vi "Length_4.vi"() -> ()   [LabVIEW 2020]
uses:
  Support/Controls/Cmd_Mouse Popup.ctl
  Support/Controls/Clst_Initialize Input.ctl
  Support/Controls/Clst_Result inspec.ctl
  Support/Controls/Cmd_Var Data IO.ctl
  Variables/Global_Cal Info.vi
panel:
  out "최소범위":string
  in  "구분 2":string(combo) caption="재질"
  in  "구분":string(combo)="2급" caption="등급"
  out "단위":string
  out "최대범위":string
  in  "Spec 변경":bool
  in  "Random":bool
  out "Spec":string[][](table)
  out "제목":string
  out "에러 출력":errorcluster
  out "Condition":string[][](table) caption="2. 직선성 시험"
  in  "Measured":string[][](table) caption="지시편차 (μm)"
  out "Load?":bool
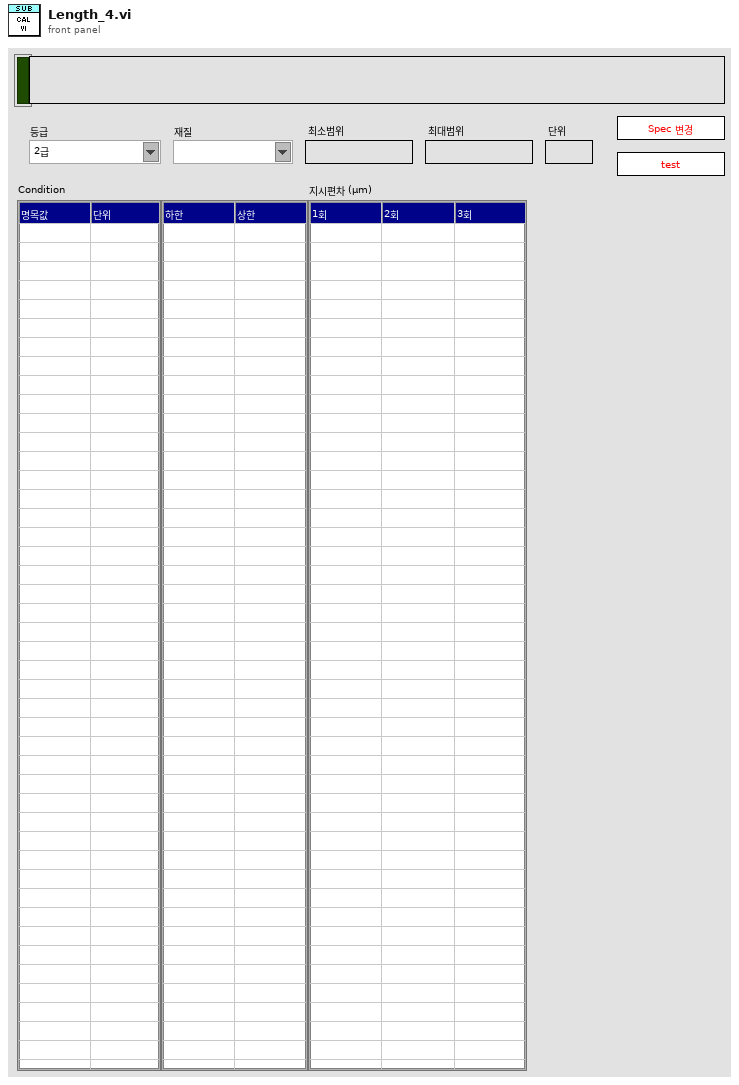
[diagram p1: front panel]
types:
  T1 = typedef "Cmd_Mouse Popup.ctl" = enum16{"활성화", "메뉴선택"}
  T2 = cluster{"Shift":bool, "Ctrl":bool, "Alt":bool, "Cmd":bool, "Opt":bool}
  T3 = typedef "Clst_Initialize Input.ctl" = cluster{"Initialize 1":cluster{"Condition":refnum<vi>[], "Spec":refnum<vi>[], "Measured":refnum<vi>[], "Resolution":refnum<vi>[], "Func_ext":string, "제목":refnum<vi>, "Measured_ADJ":refnum<vi>[]}, "Initialize 2":cluster{"문자열":refnum<vi>[], "콤보박스":refnum<vi>[], "링":refnum<vi>[], "열거형":refnum<vi>[], "테이블":refnum<vi>[], "여러열":refnum<vi>[], "디지털(DBL)":refnum<vi>[], "3D string":refnum<vi>[], "ctrl":refnum<vi>[], "boolean":refnum<vi>[]}}
  T4 = enum8{"Enabled", "Disabled", "Disabled and Grayed Out"}
  T5 = typedef "Clst_Result inspec.ctl" = cluster{"분해능":string, "문자열 1":string, "문자열 2":string, "숫자형 1":i32, "숫자형 2":i32, "숫자형 3":dbl, "문자배열 1D":string[], "문자배열 2D":string[][], "문자배열 3D":string[][][], "문자배열 4D":string[][][][], "불리언 1D":bool[]}
  T6 = typedef "Cmd_Var Data IO.ctl" = enum16{"Condition", "Condition Default", "Condition_Temp", "Resolution", "Resolution Default", "Resolution Old", "Spec", "Spec Default", "Spec Old", "Spec Temp", "Result", "Result2", "Result3", "Result_Temp", "Result_ADJ", "Result_ADJ2", "STD1", "STD2", "STD3", "STD4", "STD5", "STD Temp", "CMC", "CMC Default"}
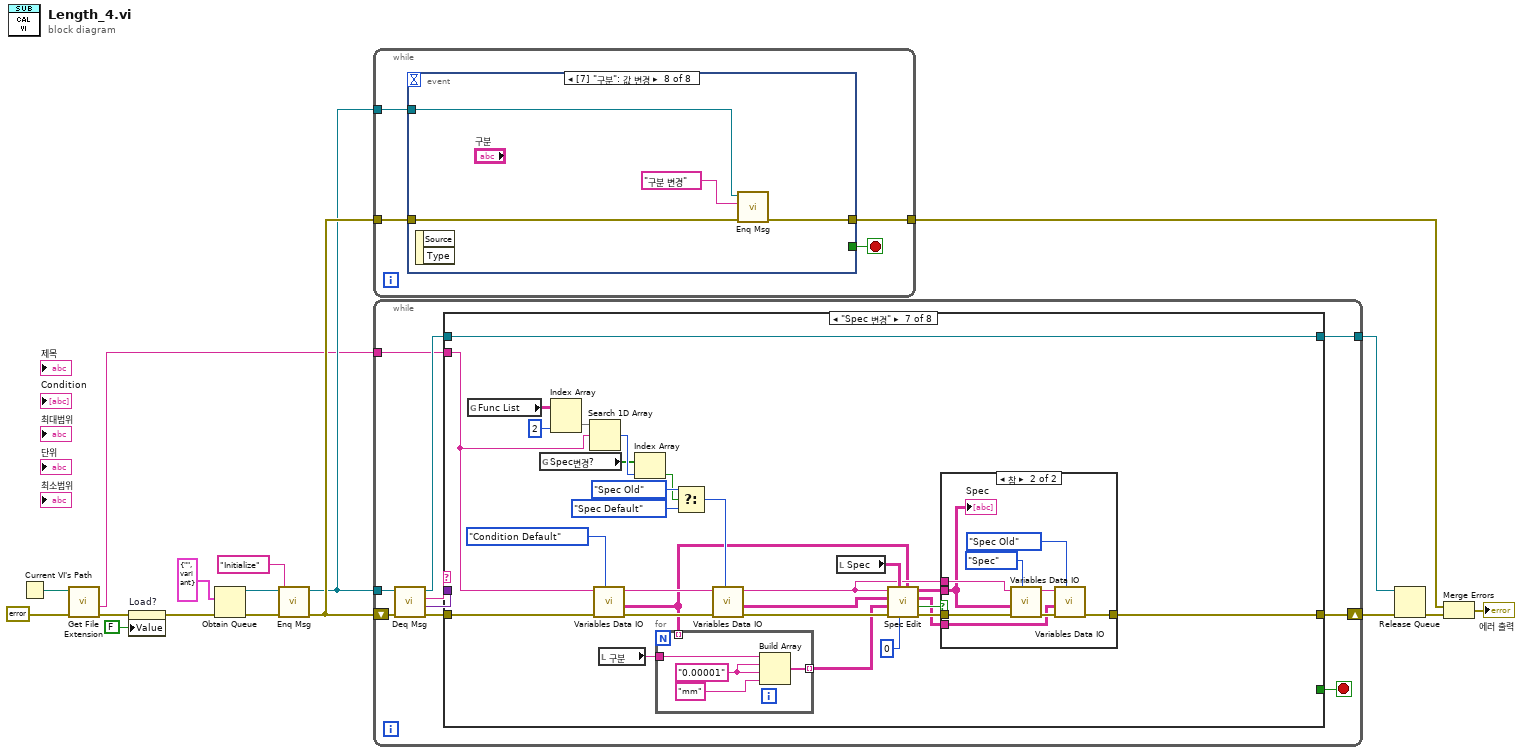
[diagram p0: block diagram]
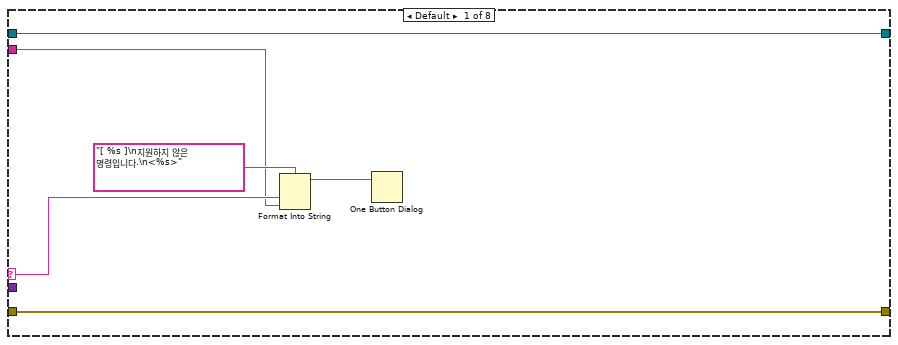
[diagram p2: hidden frame]
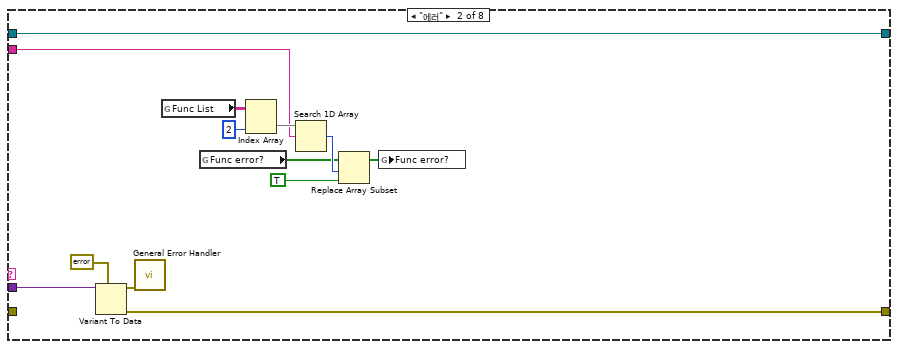
[diagram p3: hidden frame]
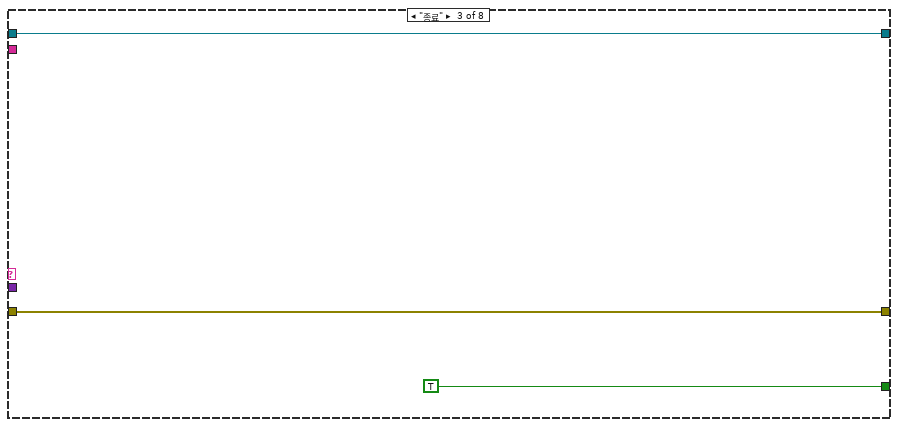
[diagram p4: hidden frame]
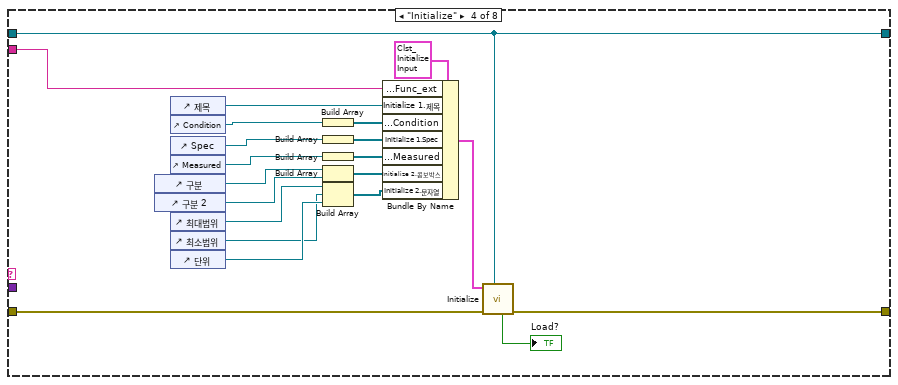
[diagram p5: hidden frame]
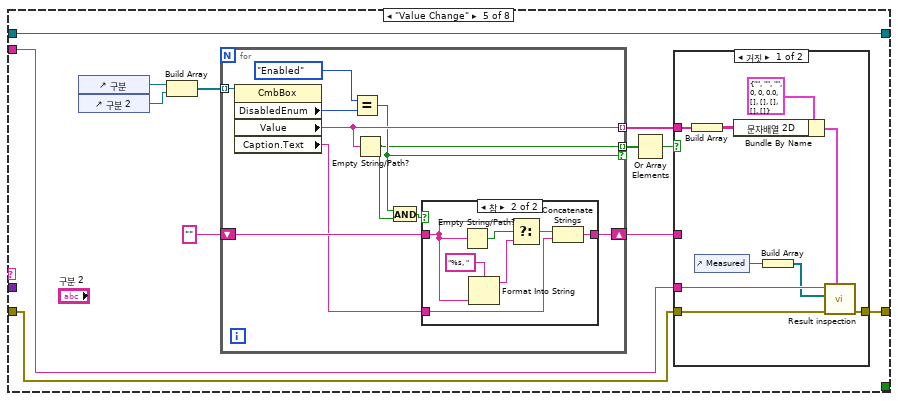
[diagram p6: hidden frame]
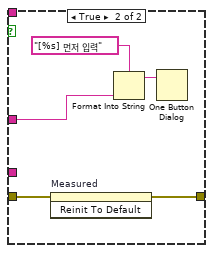
[diagram p8: hidden frame]
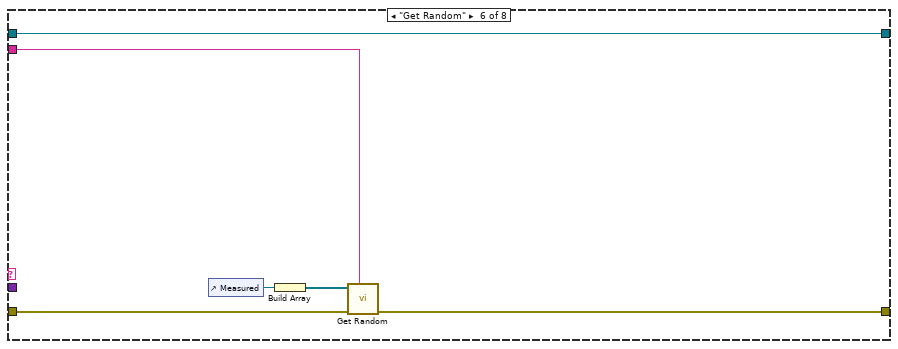
[diagram p9: hidden frame]
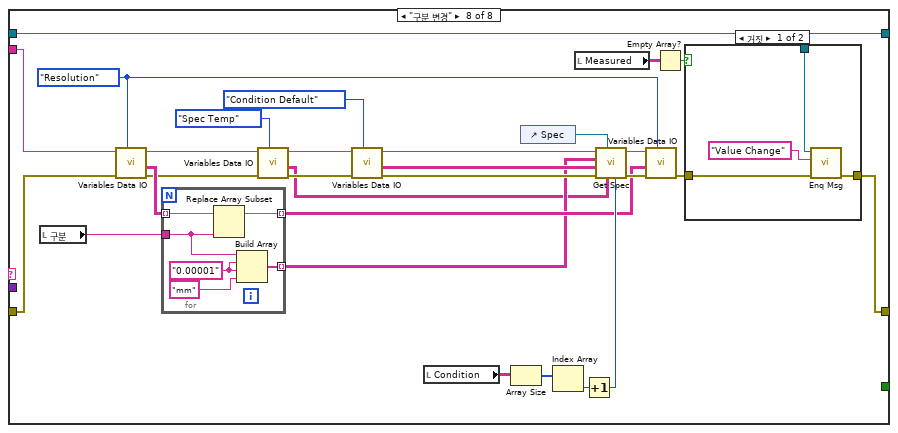
[diagram p11: hidden frame]
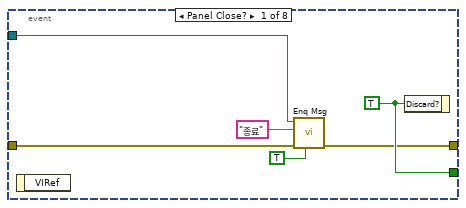
[diagram p13: hidden frame]
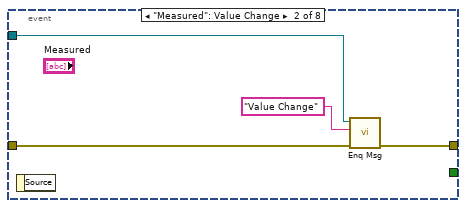
[diagram p14: hidden frame]
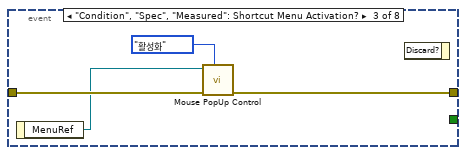
[diagram p15: hidden frame]
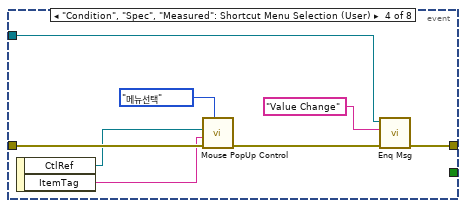
[diagram p16: hidden frame]
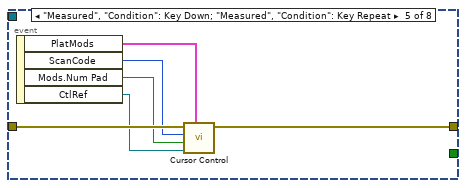
[diagram p17: hidden frame]
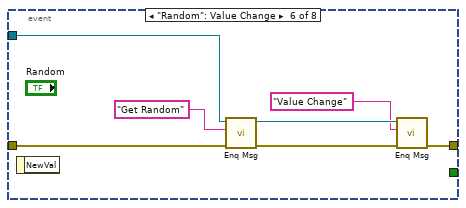
[diagram p18: hidden frame]
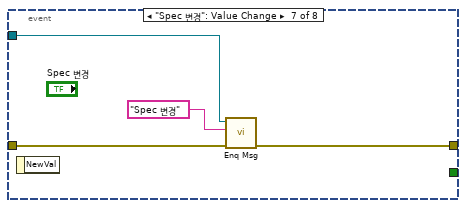
[diagram p19: hidden frame]
diagram:
  n1 = Current VI's Path() -> (path=w5:path)
  n2 = call <vilib>:"Get File Extension.vi"("error in (no error)"=errorcluster {"status"=FALSE, "code"=0, "source"=""} ("에러 상수"), "file"=w5) -> ("error out"=w3:errorcluster, "filename without extension"=w4:string)  [unwired: 5 in, 3 out]
  n3 = property on="Load?" class="Bool (엄격한)"(error in=w3, "Value"=FALSE ("Load?")) -> (error out=w2:errorcluster)  [unwired: 1 in, 1 out]
  n4 = Obtain Queue(element data type=cluster{"메세지":string, "값":variant} {"메세지"="", "값"=variant} ("Message Cluster"), error in (no error)=w2) -> (queue out=w14:refnum<queue>, error out=w16:errorcluster)  [unwired: 3 in, 1 out]
  n5 = call "Enq Msg.vi"("에러 입력(에러 없음)"=w16, "메세지"="Initialize", "큐 입력"=w14) -> ("에러 출력"=w15:errorcluster, "큐 출력"=w12:refnum<queue>)  [unwired: 7 in]
  n6 = while {
    tunnel: w15 -> [w19]
    tunnel: w12 -> [w20]
    tunnel: [w18] -> w9
    stop <- w21 stop-if-true
    n7 = event shown="[7] \"구분\": 값 변경" {
      selector: _ -> [_ _ _ _ _ _ _ _]
      dyn-events: _ -> [_ _ _ _ _ _ _ _]
      timeout: _ -> [_ _ _ _ _ _ _ _]
      tunnel: [w27 _ _ _ _ _ _ _] -> w21
      tunnel: w20 -> [w25 w31 _ w36 _ w54 w58 w61]
      tunnel: w19 -> [w26 w29 w35 w43 w49 w55 w59 w63]
      tunnel: [w23 w30 w34 w37 w48 w50 w57 w62] -> w18
      event Panel Close? {
        w27 = TRUE ("버림?")
        n8 = event-data() -> ()  [unwired: 1 in, 1 out]
        n9 = call "Enq Msg.vi"("우선순위 메시지?"=TRUE, "에러 입력(에러 없음)"=w26, "메세지"="종료", "큐 입력"=w25) -> ("에러 출력"=w23:errorcluster)  [unwired: 6 in, 1 out]
        n10 = event-data("Discard?"=w27) -> ()  [unwired: 1 in, 1 out]
      }
      event "Measured": Value Change {
        n11 = event-data() -> ()  [unwired: 1 in, 1 out]
        n12 = call "Enq Msg.vi"("에러 입력(에러 없음)"=w29, "메세지"="Value Change", "큐 입력"=w31) -> ("에러 출력"=w30:errorcluster)  [unwired: 7 in, 1 out]
      }
      event "Condition", "Spec", "Measured": Shortcut Menu Activation? {
        n13 = event-data() -> ("MenuRef"=w33:refnum<k9>)  [unwired: 1 in]
        n14 = call "Mouse PopUp Control.vi"("type"=Cmd_Mouse_Popup."활성화", "error in"=w35, "메뉴 참조"=w33) -> ("error out"=w34:errorcluster)  [unwired: 8 in]
        n15 = event-data() -> ()  [unwired: 2 in, 1 out]
      }
      event "Condition", "Spec", "Measured": Shortcut Menu Selection (User) {
        n16 = event-data() -> ("CtlRef"=w41:refnum<vi>, "ItemTag"=w40:string)  [unwired: 1 in]
        n17 = call "Mouse PopUp Control.vi"("type"=Cmd_Mouse_Popup."메뉴선택", "error in"=w43, "아이템 태그"=w40, "Tbl 참조 번호"=w41) -> ("error out"=w38:errorcluster)  [unwired: 7 in]
        n18 = call "Enq Msg.vi"("에러 입력(에러 없음)"=w38, "메세지"="Value Change", "큐 입력"=w36) -> ("에러 출력"=w37:errorcluster)  [unwired: 7 in, 1 out]
      }
      event "Measured", "Condition": Key Down; "Measured", "Condition": Key Repeat {
        n19 = event-data() -> ("PlatMods"=w44:T2, "ScanCode"=w47:i16, "Mods.Num Pad"=w46:bool, "CtlRef"=w45:refnum<vi>)  [unwired: 1 in]
        n20 = call "Cursor Control.vi"("플랫폼 조합키"=w44, "참조"=w45, "Num Pad"=w46, "ScanCode"=w47, "error in"=w49) -> ("error out"=w48:errorcluster)  [unwired: 5 in, 1 out]
      }
      event "Random": Value Change {
        n21 = event-data() -> ()  [unwired: 1 in, 1 out]
        n22 = call "Enq Msg.vi"("에러 입력(에러 없음)"=w55, "메세지"="Get Random", "큐 입력"=w54) -> ("에러 출력"=w53:errorcluster, "큐 출력"=w52:refnum<queue>)  [unwired: 7 in]
        n23 = call "Enq Msg.vi"("에러 입력(에러 없음)"=w53, "메세지"="Value Change", "큐 입력"=w52) -> ("에러 출력"=w50:errorcluster)  [unwired: 7 in, 1 out]
      }
      event "Spec 변경": Value Change {
        n24 = event-data() -> ()  [unwired: 1 in, 1 out]
        n25 = call "Enq Msg.vi"("에러 입력(에러 없음)"=w59, "메세지"="Spec 변경", "큐 입력"=w58) -> ("에러 출력"=w57:errorcluster)  [unwired: 7 in, 1 out]
      }
      event "구분": Value Change {
        n26 = event-data() -> ()  [unwired: 1 in, 2 out]
        n27 = call "Enq Msg.vi"("에러 입력(에러 없음)"=w63, "메세지"="구분 변경", "큐 입력"=w61) -> ("에러 출력"=w62:errorcluster)  [unwired: 7 in, 1 out]
      }
    }
  }
  n28 = while {
    shift-right: [w74] -> w11
    shift-left: w15 -> [w73]
    tunnel: w12 -> [w71]
    tunnel: [w66] -> w10
    tunnel: w4 -> [w65]
    stop <- w67 stop-if-true
    n29 = call "Deq Msg.vi"("에러 입력(에러 없음)"=w73, "큐 입력"=w71) -> ("에러 출력"=w72:errorcluster, "값"=w68:variant, "메세지"=w70:string, "큐 출력"=w69:refnum<queue>)  [unwired: 6 in]
    n30 = case shown="\"Spec 변경\"" w70 {
      selector: w70 -> [w76 _ _ _ _ _ _ _]
      tunnel: w72 -> [w80 _ w96 w117 w126 w163 w171 w219]
      tunnel: [w80 w90 w96 w108 w128 w164 w191 w227] -> w74
      tunnel: w69 -> [w79 w89 w94 w104 w129 w167 w195 w226]
      tunnel: w68 -> [_ w91 _ _ _ _ _ _]
      tunnel: [_ _ TRUE ("버림?") _ _ _ _ _] -> w67
      tunnel: [w79 w89 w94 w104 w129 w167 w195 w226] -> w66
      tunnel: w65 -> [w75 w81 _ w105 w127 w162 w172 w220]
      frame Default {
        n31 = Format Into String(format string="[ %s ]\n지원하지 않은 명령입니다.\n<%s>" ("메시지"), w76, w75) -> (resulting string=w77:string)  [unwired: 2 in, 1 out]
        n32 = One Button Dialog(message=w77) -> ()  [unwired: 1 in, 1 out]
      }
      frame "에러" {
        n33 = Variant To Data(type=errorcluster {"status"=FALSE, "code"=0, "source"=""} ("에러 출력"), Variant=w91) -> (data=w93:errorcluster, error out=w90:errorcluster)  [unwired: 1 in]
        n34 = call <vilib>:"General Error Handler.vi"("error in (no error)"=w93) -> ()  [unwired: 10 in, 5 out]
        n35 = global read "Global_Cal Info.vi" "Func List"() -> (w83:string[][])
        n36 = global read "Global_Cal Info.vi" "Func error?"() -> (w86:bool[])
        n37 = Index Array(array=w83, index (col)=2 ("비활성화된 인덱스 (열)")) -> (element=w84:string[])  [unwired: 1 in]
        n38 = Search 1D Array(1D array=w84, element=w81) -> (index of element=w87:i32)  [unwired: 1 in]
        n39 = Replace Array Subset(array=w86, new element=TRUE ("새 원소/부분배열"), index=w87) -> (w88:bool[])
        n40 = global write "Global_Cal Info.vi" "Func error?"(w88) -> ()
      }
      frame "종료" {
      }
      frame "Initialize" {
        n41 = control-ref of="구분"() -> (w100:refnum<vi>)
        n42 = control-ref of="구분 2"() -> (w99:refnum<vi>)
        n43 = control-ref of="제목"() -> (w109:refnum<vi>)
        n44 = control-ref of="Condition"() -> (w114:refnum<vi>)
        n45 = control-ref of="Spec"() -> (w107:refnum<vi>)
        n46 = control-ref of="Measured"() -> (w111:refnum<vi>)
        n47 = control-ref of="최대범위"() -> (w101:refnum<vi>)
        n48 = control-ref of="최소범위"() -> (w97:refnum<vi>)
        n49 = control-ref of="단위"() -> (w103:refnum<vi>)
        n50 = Build Array(w114) -> (w113:refnum<vi>[])
        n51 = Build Array(w107) -> (w106:refnum<vi>[])
        n52 = Build Array(w111) -> (w112:refnum<vi>[])
        n53 = Build Array(w100, w99) -> (w110:refnum<vi>[])
        n54 = Build Array(w101, w97, w103) -> (w102:refnum<vi>[])
        n55 = Bundle By Name(cluster=T3 {"Initialize 1"={"Condition"=[], "Spec"=[], "Measured"=[], "Resolution"=[], "Func_ext"="", "제목"=refnum, "Measured_ADJ"=[]}, "Initialize 2"={"문자열"=[], "콤보박스"=[], "링"=[], "열거형"=[], "테이블"=[], "여러열"=[], "디지털(DBL)"=[], "3D string"=[], "ctrl"=[], "boolean"=[]}} ("입력 클러스터"), "Initialize 1.Func_ext"=w105, "Initialize 1.제목"=w109, "Initialize 1.Condition"=w113, "Initialize 1.Spec"=w106, "Initialize 1.Measured"=w112, "Initialize 2.콤보박스"=w110, "Initialize 2.문자열"=w102) -> (w115:T3)
        n56 = call "Initialize.vi"("큐 입력"=w104, "error in"=w117, "입력 클러스터"=w115) -> ("error out"=w108:errorcluster, "Load?"=→"Load?":bool)  [unwired: 5 in, 2 out]
      }
      frame "Value Change" {
        n57 = control-ref of="구분"() -> (w120:refnum<vi>)
        n58 = control-ref of="구분 2"() -> (w119:refnum<vi>)
        n59 = Build Array(w120, w119) -> (w118:refnum<vi>[])
        n60 = for {
          tunnel: w118 -> [w139] mode=indexing
          tunnel: [w136] -> w123 mode=indexing
          tunnel: [w131] -> w124 mode=indexing if=w132
          shift-right: [w133] -> w122
          shift-left: "" -> [w135]
          n61 = property class="CmbBox"(reference=w139) -> ("DisabledEnum"=w137:T4, "Value"=w136:string, "Caption.Text"=w134:string)  [unwired: 1 in, 2 out]
          n62 = Equal?(x=T4."Enabled" ("DisabledEnum"), y=w137) -> (x = y?=w132:bool)
          n63 = Empty String/Path?(string/path=w136) -> (empty?=w131:bool)
          n64 = And(x=w132, y=w131) -> (x .and. y?=w130:bool)
          n65 = case shown="참" w130 {
            tunnel: w135 -> [w140 w143]
            tunnel: w134 -> [_ w142]
            tunnel: [w140 w141] -> w133
            frame False {
            }
            frame True {
              n66 = Empty String/Path?(string/path=w143) -> (empty?=w147:bool)
              n67 = Format Into String(format string="%s, " ("포맷 문자열"), w143) -> (resulting string=w145:string)  [unwired: 2 in, 1 out]
              n68 = Select(t=w143, s=w147, f=w145) -> (s? t:f=w144:string)
              n69 = Concatenate Strings(w144, w142) -> (w141:string)
            }
          }
        }
        n70 = Or Array Elements(Boolean array=w124) -> (logical OR=w125:bool)
        n71 = case shown="거짓" w125 {
          tunnel: [w156 w158] -> w128
          tunnel: w127 -> [w155 _]
          tunnel: w126 -> [w150 w159]
          tunnel: w123 -> [w148 _]
          tunnel: w122 -> [_ w157]
          frame False {
            n72 = Build Array(w148) -> (w149:string[][])
            n73 = control-ref of="Measured"() -> (w154:refnum<vi>)
            n74 = Bundle By Name(cluster=T5 {"분해능"="", "문자열 1"="", "문자열 2"="", "숫자형 1"=0, "숫자형 2"=0, "숫자형 3"=0.0, "문자배열 1D"=[], "문자배열 2D"=[], "문자배열 3D"=[], "문자배열 4D"=[], "불리언 1D"=[]} ("입력 클러스터"), "문자배열 2D"=w149) -> (w151:T5)
            n75 = Build Array(w154) -> (w153:refnum<vi>[])
            n76 = call "Result inspection.vi"("입력 클러스터"=w151, "error in"=w150, "Ref. Data (Inspection)"=w153, "Func ext"=w155) -> ("error out"=w156:errorcluster)  [unwired: 4 in, 3 out]
          }
          frame True {
            n77 = invoke on="Measured" class="Tbl (엄격한)" method="Reinit To Default"(error in=w159) -> (error out=w158:errorcluster)  [unwired: 2 in, 2 out]
            n78 = Format Into String(format string="[%s] 먼저 입력" ("포맷 문자열"), w157) -> (resulting string=w160:string)  [unwired: 2 in, 1 out]
            n79 = One Button Dialog(message=w160) -> ()  [unwired: 1 in, 1 out]
          }
        }
      }
      frame "Get Random" {
        n80 = control-ref of="Measured"() -> (w166:refnum<vi>)
        n81 = Build Array(w166) -> (w165:refnum<vi>[])
        n82 = call "Get Random.vi"("Func_Ext"=w162, "에러 입력"=w163, "Meas"=w165) -> ("에러 출력"=w164:errorcluster)  [unwired: 7 in, 1 out]
      }
      frame "Spec 변경" {
        n83 = global read "Global_Cal Info.vi" "Func List"() -> (w181:string[][])
        n84 = global read "Global_Cal Info.vi" "Spec변경?"() -> (w177:bool[])
        n85 = Index Array(array=w181, index (col)=2 ("비활성화된 인덱스 (열)")) -> (element=w179:string[])  [unwired: 1 in]
        n86 = Search 1D Array(1D array=w179, element=w172) -> (index of element=w178:i32)  [unwired: 1 in]
        n87 = call "Variables Data IO.vi"("Select"=Cmd_Var_Data_IO."Condition Default", "error in"=w171, "Func_ext"=w172) -> ("error out"=w175:errorcluster, "Data Out"=w168:string[][], "Func_ext Out"=w174:string)  [unwired: 6 in]
        n88 = local read "구분"() -> (w170:string)
        n89 = Index Array(array=w177, index=w178) -> (element=w182:bool)
        n90 = for {
          tunnel: [w197] -> w169 mode=indexing
          tunnel: w170 -> [w196]
          tunnel: w168 -> [_] mode=indexing
          w199 = "0.00001" ("새 원소/부분배열")
          n91 = Build Array(w196, w199, w199, "mm" ("새 원소/부분배열")) -> (w197:string[])
        }
        n92 = Select(t=Cmd_Var_Data_IO."Spec Old" ("Select"), s=w182, f=Cmd_Var_Data_IO."Spec Default" ("Select")) -> (s? t:f=w176:T6)
        n93 = call "Variables Data IO.vi"("Select"=w176, "error in"=w175, "Func_ext"=w174) -> ("error out"=w190:errorcluster, "Data Out"=w185:string[][], "Func_ext Out"=w186:string)  [unwired: 6 in]
        n94 = local read "Spec"() -> (w187:string[][])
        n95 = call "Spec Edit.vi"("Condition"=w168, "열번호(기준값)"=0, "Spec Value"=w187, "에러 입력(에러 없음)"=w190, "Resolution"=w169, "Spec Default"=w185, "Func_ext"=w186) -> ("에러 출력"=w192:errorcluster, "변경?"=w193:bool, "Spec Default out"=w189:string[][], "Spec 출력"=w194:string[][])  [unwired: 1 in]
        n96 = case shown="참" w193 {
          tunnel: w194 -> [_ w206]
          tunnel: w192 -> [w200 w209]
          tunnel: [w200 w204] -> w191
          tunnel: w186 -> [_ w207]
          tunnel: w189 -> [_ w202]
          frame False {
          }
          frame True {
            n97 = call "Variables Data IO.vi"("Select"=Cmd_Var_Data_IO."Spec", "error in"=w209, "Data In"=w206, "Func_ext"=w207) -> ("error out"=w205:errorcluster, "Func_ext Out"=w203:string)  [unwired: 5 in, 1 out]
            n98 = call "Variables Data IO.vi"("Select"=Cmd_Var_Data_IO."Spec Old", "error in"=w205, "Data In"=w202, "Func_ext"=w203) -> ("error out"=w204:errorcluster)  [unwired: 5 in, 2 out]
            "Spec" <- w206
          }
        }
      }
      frame "구분 변경" {
        w230 = Cmd_Var_Data_IO."Resolution" ("Select")
        n99 = local read "구분"() -> (w211:string)
        n100 = call "Variables Data IO.vi"("Select"=w230, "error in"=w219, "Func_ext"=w220) -> ("error out"=w217:errorcluster, "Data Out"=w229:string[][], "Func_ext Out"=w216:string)  [unwired: 6 in]
        n101 = for {
          tunnel: w211 -> [w245]
          tunnel: [w249] -> w214 mode=indexing
          tunnel: w229 -> [w248] mode=indexing
          tunnel: [w244] -> w212 mode=indexing
          w247 = "0.00001" ("새 원소/부분배열")
          n102 = Replace Array Subset(array=w248, new element=w245) -> (w249:string[])  [unwired: 1 in]
          n103 = Build Array(w245, w247, w247, "mm" ("새 원소/부분배열")) -> (w244:string[])
        }
        n104 = call "Variables Data IO.vi"("Select"=Cmd_Var_Data_IO."Spec Temp", "error in"=w217, "Func_ext"=w216) -> ("error out"=w221:errorcluster, "Data Out"=w210:string[][], "Func_ext Out"=w222:string)  [unwired: 6 in]
        n105 = call "Variables Data IO.vi"("Select"=Cmd_Var_Data_IO."Condition Default", "error in"=w221, "Func_ext"=w222) -> ("error out"=w218:errorcluster, "Data Out"=w215:string[][], "Func_ext Out"=w213:string)  [unwired: 6 in]
        n106 = local read "Condition"() -> (w236:string[][])
        n107 = Array Size(array=w236) -> (size(s)=w235:i32[])
        n108 = control-ref of="Spec"() -> (w238:refnum<vi>)
        n109 = Index Array(array=w235) -> (element=w233:i32)  [unwired: 1 in]
        n110 = local read "Measured"() -> (w225:string[][])
        n111 = Increment(x=w233) -> (x+1=w223:i32)
        n112 = call "Get Spec.vi"("NumRows"=w223, "Spec in"=w210, "Spec Ref."=w238, "error in"=w218, "Condition in"=w215, "Resolution in"=w212, "Func_ext"=w213) -> ("error out"=w231:errorcluster, "Func_ext Out"=w232:string)  [unwired: 3 out]
        n113 = call "Variables Data IO.vi"("Select"=w230, "error in"=w231, "Data In"=w214, "Func_ext"=w232) -> ("error out"=w228:errorcluster)  [unwired: 5 in, 2 out]
        n114 = Empty Array?(array=w225) -> (empty?=w224:bool)
        n115 = case shown="거짓" w224 {
          tunnel: w228 -> [w241 w243]
          tunnel: [w240 w243] -> w227
          tunnel: w226 -> [w239 _]
          frame False {
            n116 = call "Enq Msg.vi"("에러 입력(에러 없음)"=w241, "메세지"="Value Change", "큐 입력"=w239) -> ("에러 출력"=w240:errorcluster)  [unwired: 7 in, 1 out]
          }
          frame True {
          }
        }
      }
    }
  }
  n117 = Release Queue(queue=w10, error in (no error)=w11) -> (error out=w8:errorcluster)  [unwired: 1 in, 2 out]
  n118 = Merge Errors(w9, w8) -> (→"에러 출력":errorcluster)
